vi "Sub_FFT_get_freq_components.vi"(0 "Prior Frequency Estimate (Feed forward)":dbl, 1 "ACC Signal":dbl[](array[numeric]), 2 "Experimental Results":T2, 3 "Setup Parameters":T4, 4 "Beam frequency params":T3, 5 "Use Top N freq components":i32=5 min=1 max=50 step=1, 6 "Frequency selection method":T1(ring), 7 "Slop factor (Feed forward)":dbl=1.0, 9 "Bound to 1st Frequency":bool=TRUE) -> (10 "Windowed X (out)":dbl[](array[numeric]), 16 "Real freq comp (out)":dbl[](array[numeric]), 20 "Next Frequency Estimate":dbl, 21 "Low Energy":bool, 27 "Slop factor (Feed back)":dbl=1.0)   [LabVIEW 2021]
uses:
  <vilib>/Analysis/4window.llb/Hanning Window (DBL).vi
  <vilib>/Analysis/5stat.llb/RMS (DBL).vi
  <vilib>/Analysis/2dsp.llb/Real FFT.vi
  d4458743-e843-49c5-a9b9-3479e78049c0.vi
  <vilib>/Analysis/4window.llb/AllCosWindow (DBL).vi
  <vilib>/Analysis/NI_AALPro.lvlib
panel:
  out "top n freq":dbl[](array[numeric])
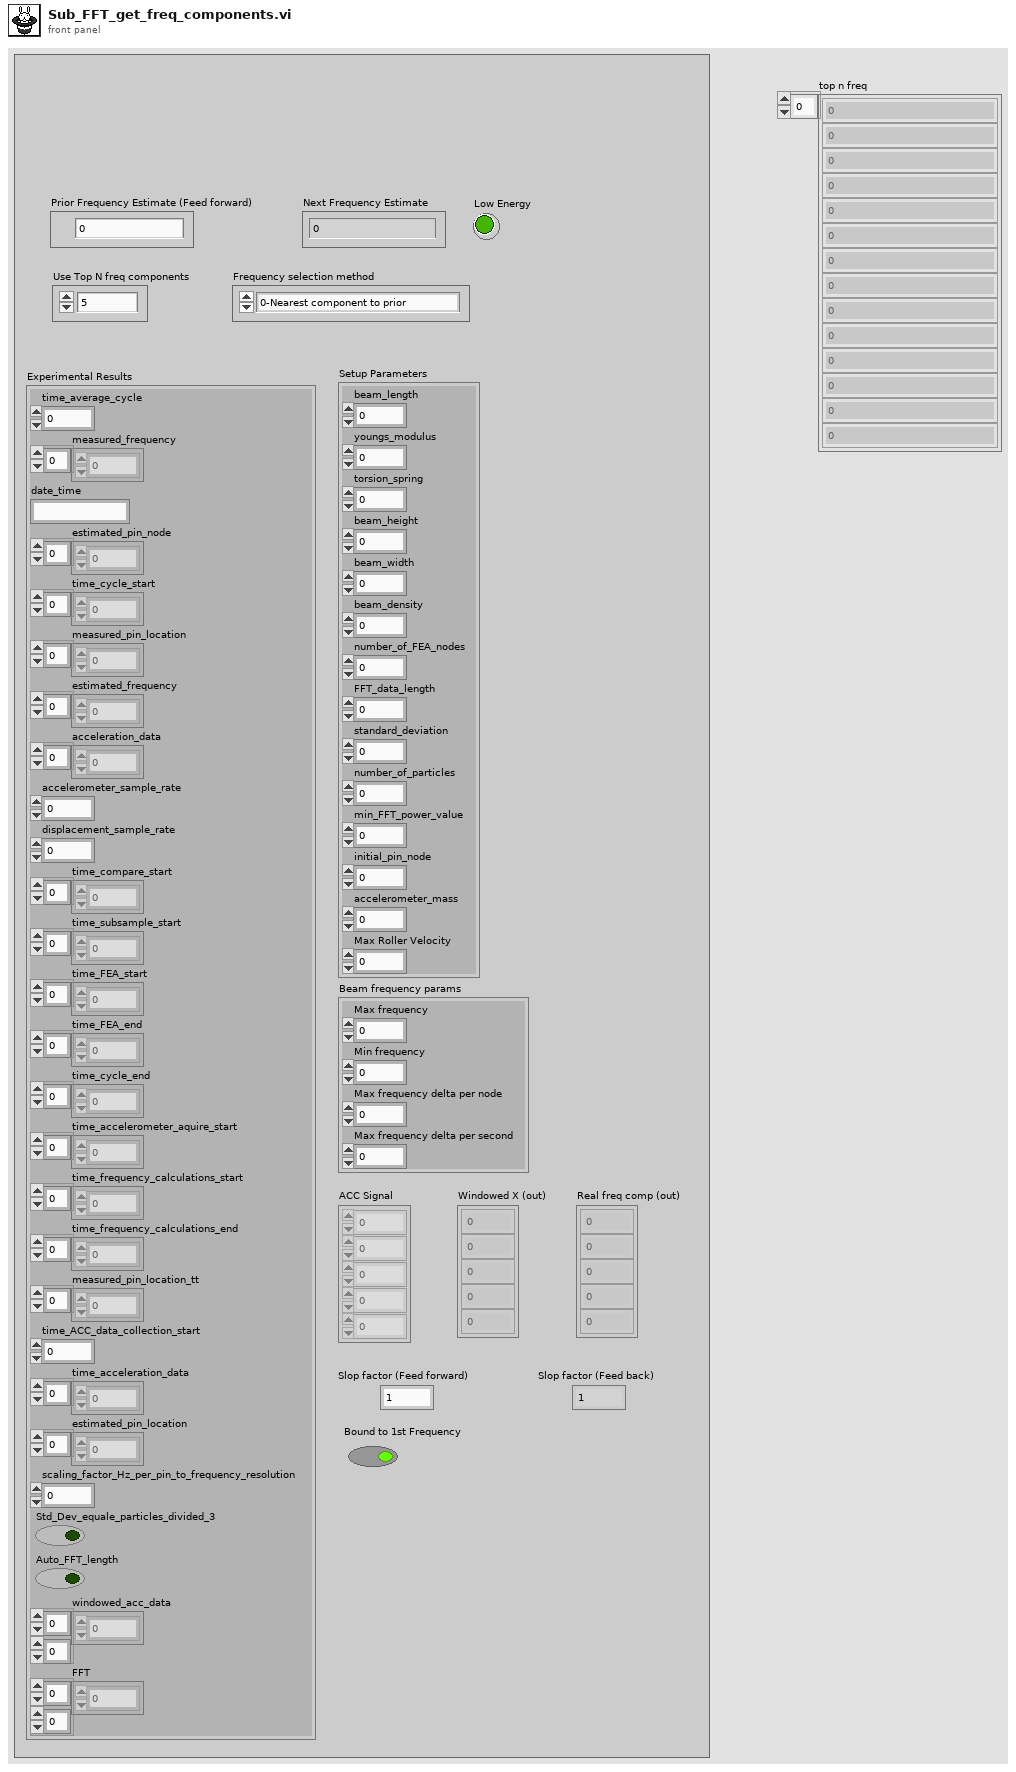
[diagram p1: front panel]
types:
  T1 = enum16{"0-Nearest component to prior ", "1-Coerce maximum differential", "2-Average with nearest component", "3-Top by power", "4-Lowest major component", "5-Average with lowest component", "6-???"}
  T2 = cluster{"time_average_cycle":dbl, "measured_frequency":dbl[], "date_time":string, "estimated_pin_node":i32[], "time_cycle_start":dbl[], "measured_pin_location":dbl[], "estimated_frequency":dbl[], "acceleration_data":dbl[], "accelerometer_sample_rate":dbl, "displacement_sample_rate":dbl, "time_compare_start":dbl[], "time_subsample_start":dbl[], "time_FEA_start":dbl[], "time_FEA_end":dbl[], "time_cycle_end":dbl[], "time_accelerometer_aquire_start":dbl[], "time_frequency_calculations_start":dbl[], "time_frequency_calculations_end":dbl[], "measured_pin_location_tt":dbl[], "time_ACC_data_collection_start":dbl, "time_acceleration_data":dbl[], "estimated_pin_location":dbl[], "scaling_factor_Hz_per_pin_to_frequency_resolution":dbl, "Std_Dev_equale_particles_divided_3":bool, "Auto_FFT_length":bool, "windowed_acc_data":dbl[][], "FFT":dbl[][]}
  T3 = cluster{"Max frequency":dbl, "Min frequency":dbl, "Max frequency delta per node":dbl, "Max frequency delta per second":dbl}
  T4 = cluster{"beam_length":dbl, "youngs_modulus":dbl, "torsion_spring":dbl, "beam_height":dbl, "beam_width":dbl, "beam_density":dbl, "number_of_FEA_nodes":i32, "FFT_data_length":i32, "standard_deviation":dbl, "number_of_particles":i32, "min_FFT_power_value":dbl, "initial_pin_node":i32, "accelerometer_mass":dbl, "Max Roller Velocity":dbl}
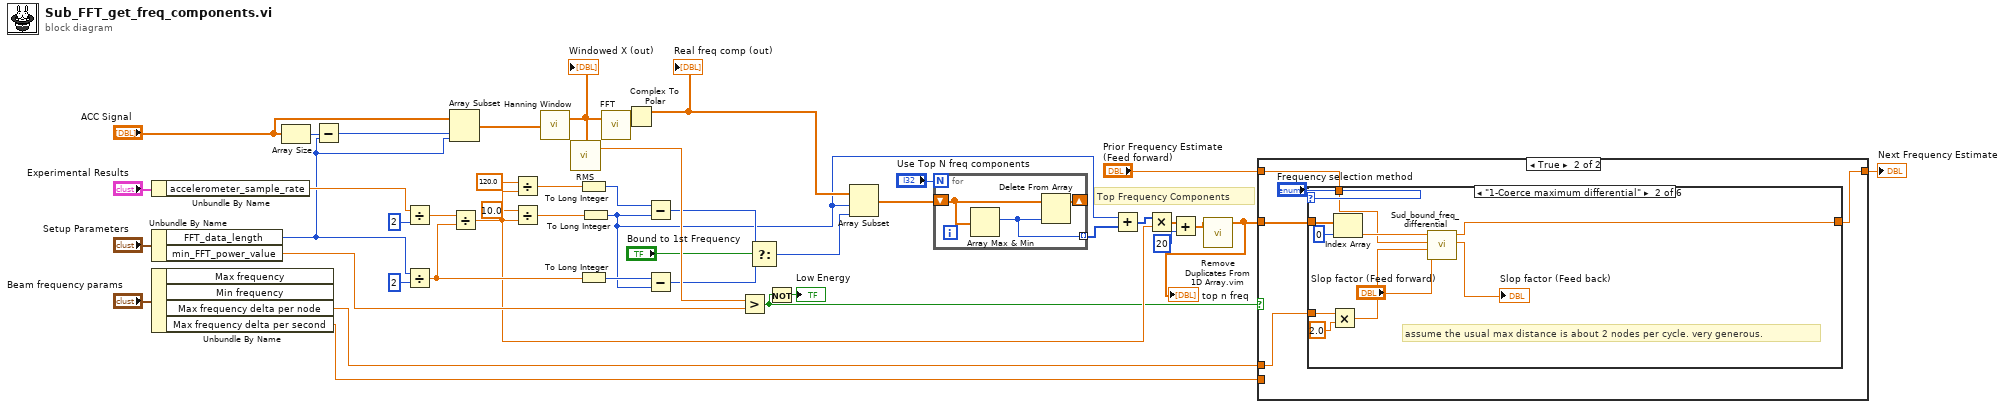
[diagram p0: block diagram]
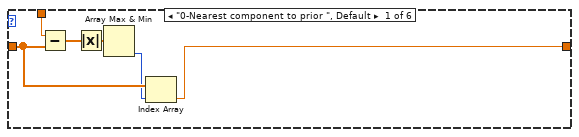
[diagram p3: hidden frame]
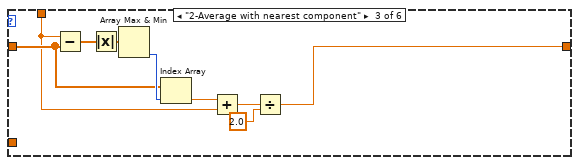
[diagram p4: hidden frame]
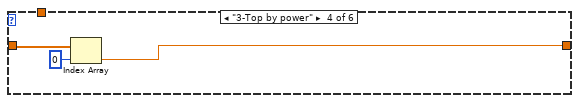
[diagram p5: hidden frame]
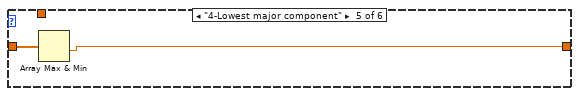
[diagram p6: hidden frame]
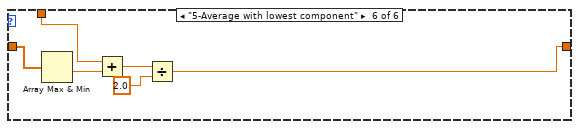
[diagram p7: hidden frame]
diagram:
  # "Top Frequency Components"
  n1 = Unbundle By Name("Experimental Results") -> ("accelerometer_sample_rate"=w44:dbl)
  n2 = Unbundle By Name("Setup Parameters") -> ("FFT_data_length"=w43:i32, "min_FFT_power_value"=w42:dbl)
  n3 = Unbundle By Name("Beam frequency params") -> ("Max frequency delta per node"=w9:dbl, "Max frequency delta per second"=w8:dbl)  [unwired: 2 out]
  n4 = Array Size(array="ACC Signal") -> (size(s)=w32:i32)
  n5 = Subtract(x=w32, y=w43) -> (x-y=w33:i32)
  n6 = Divide(x=w44, y=2) -> (x/y=w30:dbl)
  n7 = Divide(x=w43, y=2) -> (x/y=w31:dbl)
  n8 = Array Subset(array="ACC Signal", index=w33, length=w43) -> (w34:dbl[])
  n9 = Divide(x=w30, y=w31) -> (x/y=w15:dbl)
  n10 = Divide(x=120.0, y=w15) -> (x/y=w35:dbl)
  n11 = Divide(x=10.0, y=w15) -> (x/y=w27:dbl)
  n12 = call-poly <vilib>:"Hanning Window.vi"("X"=w34) -> ("Windowed X"=w23:dbl[])  [unwired: 1 out]
  "Windowed X (out)" <- w23
  n13 = call-poly <vilib>:"RMS.vi"("X"=w23) -> ("rms value"=w41:dbl)  [unwired: 1 out]
  n14 = To Long Integer(number=w35) -> (32bit integer=w36:i32)
  n15 = To Long Integer(number=w31) -> (32bit integer=w29:i32)
  n16 = To Long Integer(number=w27) -> (32bit integer=w16:i32)
  n17 = call-poly <vilib>:"FFT.vi"("X"=w23) -> ("FFT {X}"=w28:cdb[])  [unwired: 9 in, 1 out]
  n18 = Complex To Polar(r * e^(i*theta)=w28) -> (r=w24:dbl[])  [unwired: 1 out]
  "Real freq comp (out)" <- w24
  n19 = Subtract(x=w36, y=w16) -> (x-y=w39:i32)
  n20 = Subtract(x=w29, y=w16) -> (x-y=w40:i32)
  n21 = Greater?(x=w41, y=w42) -> (0:w12:bool)
  n22 = Select(t=w39, s="Bound to 1st Frequency", f=w40) -> (s? t:f=w37:i32)
  n23 = Not(x=w12) -> (.not. x?=→"Low Energy":bool)
  n24 = Array Subset(array=w24, index=w16, length=w37) -> (w18:dbl[])
  n25 = for {
    N: "Use Top N freq components" -> [_]
    shift-right: [w46] -> _
    shift-left: w18 -> [w47]
    tunnel: [w45] -> w17 mode=indexing
    n26 = Array Max & Min(array=w47) -> (max index (indices)=w45:i32)  [unwired: 3 out]
    n27 = Delete From Array(array=w47, index=w45) -> (array with subset deleted=w46:dbl[])  [unwired: 1 in, 1 out]
  }
  n28 = Add(x=w16, y=w17) -> (x+y=w13:i32[])
  n29 = Multiply(x=w13, y=w15) -> (x*y=w5:dbl[])
  n30 = Add(x=w5, y=20) -> (x+y=w4:dbl[])
  n31 = call "Remove Duplicates From 1D Array.vim"("array"=w4) -> ("array with duplicates removed"=w6:dbl[])  [unwired: 10 in]
  "top n freq" <- w6
  n32 = case shown="True" w12 {
    tunnel: "Prior Frequency Estimate (Feed forward)" -> [w48 w52]
    tunnel: [w48 w50] -> w10
    tunnel: w6 -> [_ w51]
    tunnel: w9 -> [_ w49]
    tunnel: w8 -> [_ _]
    frame False {
    }
    frame True {
      n33 = case shown="\"1-Coerce maximum differential\"" "Frequency selection method" {
        tunnel: w52 -> [w58 w66 w73 _ _ w87]
        tunnel: w51 -> [w57 w69 w75 w81 w83 w89]
        tunnel: [w54 w62 w70 w79 w82 w84] -> w50
        tunnel: w49 -> [_ w65 _ _ _ _]
        frame "0-Nearest component to prior ", Default {
          n34 = Subtract(x=w58, y=w57) -> (x-y=w59:dbl[])
          n35 = Absolute Value(x=w59) -> (abs(x)=w56:dbl[])
          n36 = Array Max & Min(array=w56) -> (min index (indices)=w55:i32)  [unwired: 3 out]
          n37 = Index Array(array=w57, index=w55) -> (element=w54:dbl)
        }
        frame "1-Coerce maximum differential" {
          # "assume the usual max distance is about 2 nodes per cycle. very generous."
          n38 = Multiply(x=w65, y=2.0) -> (x*y=w63:dbl)
          n39 = Index Array(array=w69, index=0) -> (element=w67:dbl)
          n40 = call "Sud_bound_freq_differential.vi"("Slop factor"="Slop factor (Feed forward)", "Max delta freq"=w63, "Prior Frequency estimate"=w66, "Next Frequency estimate"=w67) -> ("Slop factor (feedback)"=→"Slop factor (Feed back)":dbl, "Next Frequency estimate (Bounded)"=w62:dbl)  [unwired: 6 in]
        }
        frame "2-Average with nearest component" {
          n41 = Subtract(x=w73, y=w75) -> (x-y=w78:dbl[])
          n42 = Absolute Value(x=w78) -> (abs(x)=w77:dbl[])
          n43 = Array Max & Min(array=w77) -> (min index (indices)=w76:i32)  [unwired: 3 out]
          n44 = Index Array(array=w75, index=w76) -> (element=w74:dbl)
          n45 = Add(x=w74, y=w73) -> (x+y=w71:dbl)
          n46 = Divide(x=w71, y=2.0 ("x+y")) -> (x/y=w70:dbl)
        }
        frame "3-Top by power" {
          n47 = Index Array(array=w81, index=0) -> (element=w79:dbl)
        }
        frame "4-Lowest major component" {
          n48 = Array Max & Min(array=w83) -> (min value=w82:dbl)  [unwired: 3 out]
        }
        frame "5-Average with lowest component" {
          n49 = Array Max & Min(array=w89) -> (min value=w88:dbl)  [unwired: 3 out]
          n50 = Add(x=w87, y=w88) -> (x+y=w86:dbl)
          n51 = Divide(x=w86, y=2.0) -> (x/y=w84:dbl)
        }
      }
    }
  }
  "Next Frequency Estimate" <- w10
